vi "lakeshore_372.vi"() -> ()   [LabVIEW 2020]
panel:
  in  "VISA Refnum in":refnum<visa-resource-name>
  in  "ID Query":string
  out "read buffer 2":string
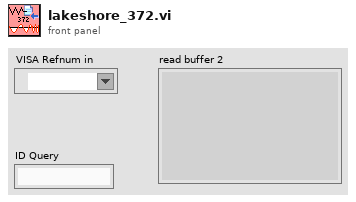
[diagram p1: front panel]
types:
  T1 = cluster{"Baud Rate":u32, "Parity":u16, "Data Bits":u16, "Stop Bits":u16, "Flow Control":u16}
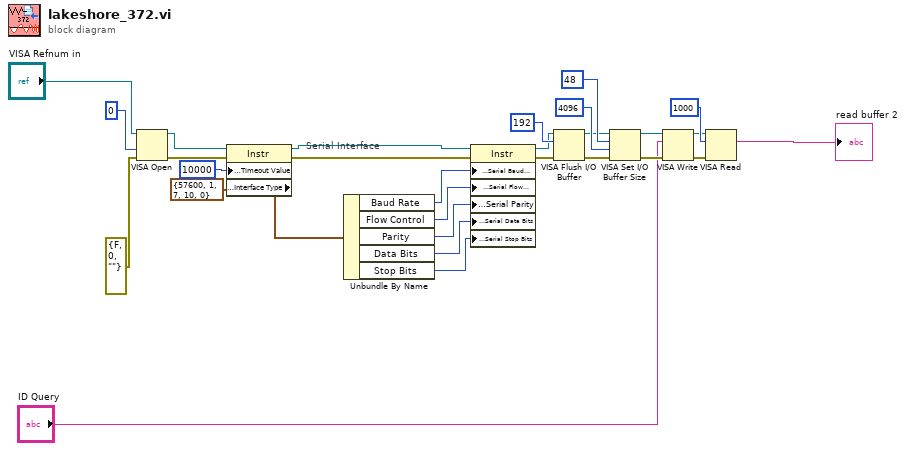
[diagram p0: block diagram]
diagram:
  # "Serial Interface"
  n1 = VISA Open(access mode=u32 0, error in (no error)=errorcluster {"status"=FALSE, "code"=0, "source"=""}, VISA resource name="VISA Refnum in") -> (VISA resource name=w3:refnum<visa-resource-name>, error out=w4:errorcluster)  [unwired: 2 in]
  n2 = property class="Instr" props=["General Settings:Timeout Value", "Interface Information:Interface Type"](reference=w3, error in=w4, "General Settings:Timeout Value"=u32 10000) -> (reference out=w5:refnum<visa-resource-name>, error out=w6:errorcluster)  [unwired: 1 out]
  n3 = Unbundle By Name(T1 {"Baud Rate"=57600, "Parity"=1, "Data Bits"=7, "Stop Bits"=10, "Flow Control"=0} ("Serial Configuration")) -> ("Baud Rate"=w18:u32, "Flow Control"=w22:u16, "Parity"=w20:u16, "Data Bits"=w19:u16, "Stop Bits"=w23:u16)
  n4 = property class="Instr"(reference=w5, error in=w6, "Serial Settings:Serial Baud Rate"=w18, "Serial Settings:Serial Flow Control"=w22, "Serial Settings:Serial Parity"=w20, "Serial Settings:Serial Data Bits"=w19, "Serial Settings:Serial Stop Bits"=w23) -> (reference out=w17:refnum<visa-resource-name>, error out=w15:errorcluster)
  n5 = VISA Flush I/O Buffer(VISA resource name=w17, mask (16)=u16 192, error in (no error)=w15) -> (VISA resource name out=w14:refnum<visa-resource-name>, error out=w16:errorcluster)
  n6 = VISA Set I/O Buffer Size(VISA resource name=w14, mask (16)=u16 48, size (4096)=u32 4096 ("size (0)"), error in (no error)=w16) -> (VISA resource name out=w28:refnum<visa-resource-name>, error out=w27:errorcluster)
  n7 = VISA Write(VISA resource name=w28, write buffer="ID Query", error in (no error)=w27) -> (VISA resource name out=w10:refnum<visa-resource-name>, error out=w9:errorcluster)  [unwired: 1 out]
  n8 = VISA Read(VISA resource name=w10, byte count=u32 1000, error in (no error)=w9) -> (read buffer=→"read buffer 2":string)  [unwired: 3 out]
